vi "GUI_THALES_images.vi"() -> ()   [LabVIEW 2013]
panel:
  out "time":dbl format="%#.0f"
  out "error out":errorcluster
  in  "error in (no error)":errorcluster
  in  "Root path":path
  in  "time between saves (seconds)":u32=10
  in  "stop":bool
  out "Booster":u8[][](graph)
  out "Preamp":u8[][](graph)
  out "Amp1":u8[][](graph)
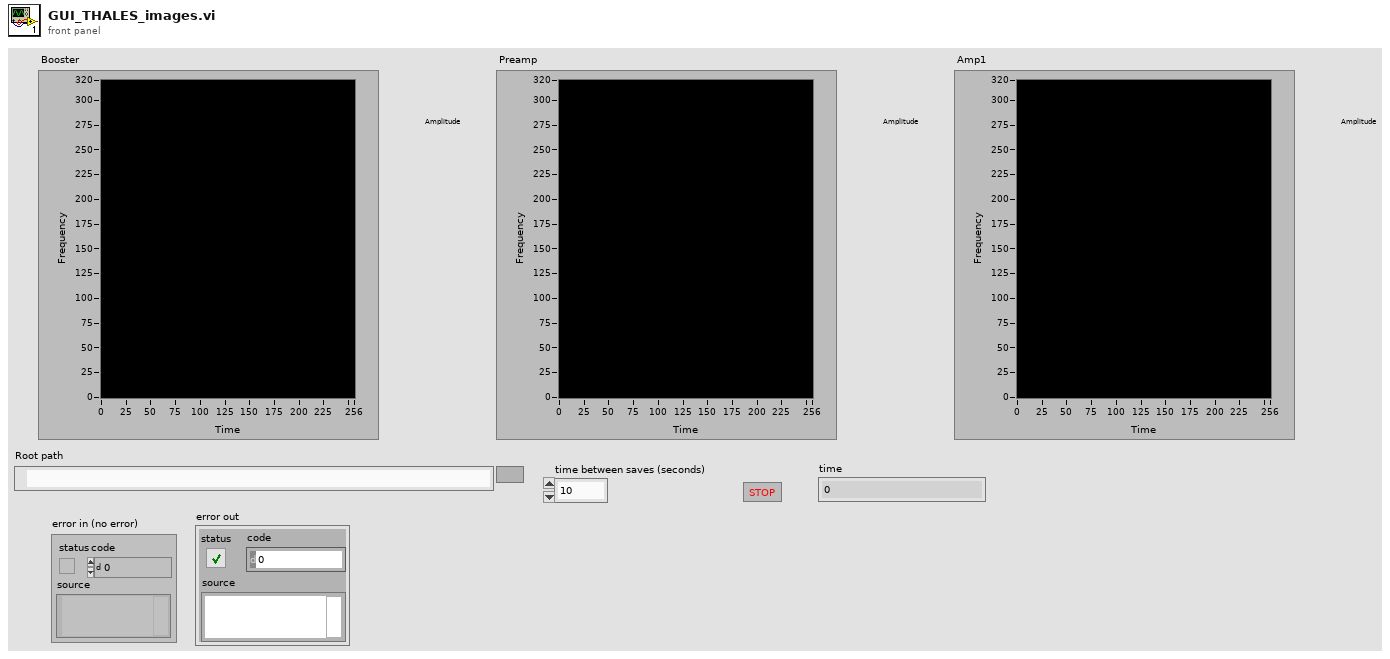
[diagram p1: front panel]
types:
  T1 = typedef "Image Type" = u32
  T2 = typedef "IMAQ Image.ctl" = refnum<image>
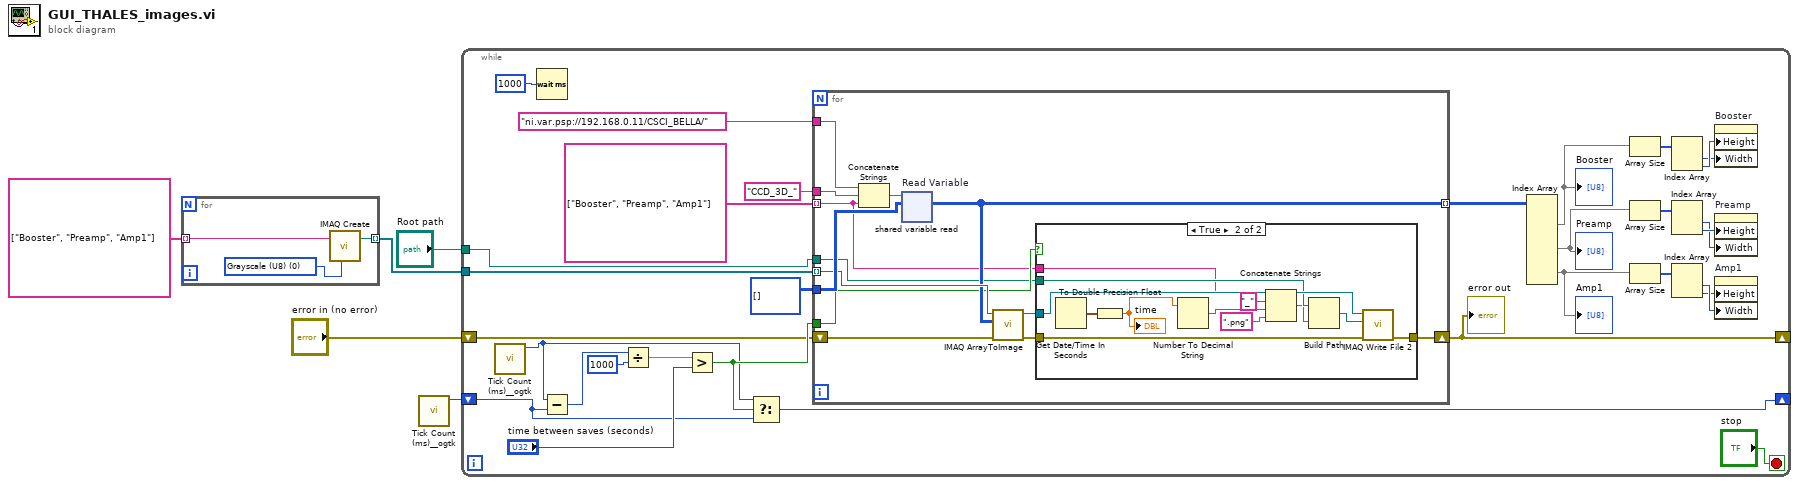
[diagram p0: block diagram]
diagram:
  n1 = for {
    tunnel: string[] ["Booster", "Preamp", "Amp1"] -> [w7] mode=indexing
    tunnel: [w6] -> w4 mode=indexing
    w8 = T1 0 items=["Grayscale (U8)", "Grayscale (I16)", "Grayscale (SGL)", "Complex (CSG)", "RGB (U32)", "HSL (U32)", "RGB (U64)", "Grayscale (U16)"] ("Image Type")
    n2 = call "IMAQ Create"("Image Name"=w7, "Image Type"=w8) -> ("New Image"=w6:T2)  [unwired: 3 in, 1 out]
  }
  n3 = call <userlib>:"Tick Count (ms)__ogtk.vi"() -> ("millisecond timer value"=w3:u32)  [unwired: 10 in, 1 out]
  n4 = while {
    tunnel: w4 -> [w20]
    shift-right: [w14] -> _
    shift-left: w3 -> [w9]
    tunnel: "Root path" -> [w13]
    shift-right: [w11] -> _
    shift-left: "error in (no error)" -> [w12]
    stop <- "stop" stop-if-true
    n5 = call <userlib>:"Tick Count (ms)__ogtk.vi"() -> ("millisecond timer value"=w10:u32)  [unwired: 10 in, 1 out]
    n6 = Wait (ms)(milliseconds to wait=u32 1000) -> ()  [unwired: 1 out]
    n7 = Subtract(x=w10, y=w9) -> (x-y=w19:u32)
    n8 = Divide(x=w19, y=u32 1000) -> (x/y=w17:dbl)
    n9 = Greater?(x=w17, y="time between saves (seconds)") -> (0:w15:bool)
    n10 = Select(t=w10, s=w15, f=w9) -> (s? t:f=w14:u32)
    n11 = for {
      tunnel: "ni.var.psp://192.168.0.11/CSCI_BELLA/" ("Var_name") -> [w52]
      tunnel: "CCD_3D_" ("Var_name") -> [w51]
      tunnel: u8[][] [] -> [w49]
      tunnel: [w47] -> w35 mode=indexing
      tunnel: string[] ["Booster", "Preamp", "Amp1"] -> [w40] mode=indexing
      tunnel: w20 -> [w48] mode=indexing
      tunnel: w15 -> [w45]
      tunnel: w13 -> [w41]
      shift-right: [w42] -> w11
      shift-left: w12 -> [w43]
      n12 = Concatenate Strings(w52, w51, w40) -> (w50:string)
      n13 = shared-variable-read "Read Variable"(w50, w49) -> (w47:u8[][])  [unwired: 1 in, 3 out]
      n14 = call "IMAQ ArrayToImage"("error in (no error)"=w43, "Image Pixels (U8)"=w47, "Image"=w48) -> ("error out"=w44:errorcluster, "Image Out"=w46:T2)  [unwired: 7 in]
      n15 = case shown="True" w45 {
        tunnel: w46 -> [_ w65]
        tunnel: w44 -> [w53 w64]
        tunnel: [w53 w63] -> w42
        tunnel: w41 -> [_ w60]
        tunnel: w40 -> [_ w55]
        frame False {
        }
        frame True {
          n16 = Get Date/Time In Seconds() -> (seconds since 1Jan1904=w62:timestamp)
          n17 = To Double Precision Float(number=w62) -> (double precision float=w61:dbl)
          "time" <- w61
          n18 = Number To Decimal String(number=w61) -> (decimal integer string=w59:string)  [unwired: 1 in]
          n19 = Concatenate Strings(w55, "_" ("string"), w59, ".png" ("string")) -> (w57:string)
          n20 = Build Path(base path=w60, name or relative path=w57) -> (appended path=w56:path)
          n21 = call-poly "IMAQ Write File 2"("error in (no error)"=w64, "File Path"=w56, "Image"=w65) -> ("error out"=w63:errorcluster)  [unwired: 7 in, 1 out]
        }
      }
    }
    "error out" <- w11
    n22 = Index Array(array=w35) -> (element #1=w32:u8[][], element #2=w29:u8[][], element #3=w21:u8[][])  [unwired: 9 in]
    "Amp1" <- w21
    "Preamp" <- w29
    "Booster" <- w32
    n23 = Array Size(array=w32) -> (size(s)=w31:i32[])
    n24 = Array Size(array=w29) -> (size(s)=w30:i32[])
    n25 = Array Size(array=w21) -> (size(s)=w28:i32[])
    n26 = Index Array(array=w31) -> (element #1=w24:i32, element #2=w25:i32)  [unwired: 2 in]
    n27 = Index Array(array=w30) -> (element #1=w22:i32, element #2=w23:i32)  [unwired: 2 in]
    n28 = Index Array(array=w28) -> (element #1=w27:i32, element #2=w26:i32)  [unwired: 2 in]
    n29 = property on="Booster" class="IntGraph (strict)"("Height"=w25, "Width"=w24) -> ()  [unwired: 2 in, 2 out]
    n30 = property on="Preamp" class="IntGraph (strict)"("Height"=w23, "Width"=w22) -> ()  [unwired: 2 in, 2 out]
    n31 = property on="Amp1" class="IntGraph (strict)"("Height"=w26, "Width"=w27) -> ()  [unwired: 2 in, 2 out]
  }
